vi "Initialize Hawkeye.vi"(0 "Repo / Workspace Folder Path":path, 1 "Generate Project for LVLib & Orphan Class":bool, 5 "LVLib / LVClass / Folder Path":path, 7 "Generate YAML Workflow from Template":bool, 9 "Generate Hawkeye Configuration from Template":bool, 12 "Generate .Hawkey File":bool) -> (4 "Status Indicator":string)   [LabVIEW 2019, in "HawkeyeToolsMenu.lvlib"]
doc: "GUI to compare LabVIEW code between currently checked out branch with any other branch or any of its commits.\n\n(c) 2024 Soliton Technologies. All rights reserved."
uses:
  HawkeyeToolsMenu.lvlib
  <vilib>/Hampel Software Engineering/Git API/Git API/GIT-api.lvclass
  <vilib>/Hampel Software Engineering/Git API/Git API/GIT-api.lvclass/GIT-api.ctl
  <vilib>/Hampel Software Engineering/Git API/Git API/Accessors/GIT-Set Working Dir.vi
  <userlib>/_OpenG.lib/file/file.llb/Valid Path - Traditional__ogtk.vi
  <userlib>/_OpenG.lib/file/file.llb/Compare Two Paths - Scalar__ogtk.vi
  <userlib>/_OpenG.lib/file/file.llb/File Exists - Scalar__ogtk.vi
  vi.lib/Hawkeye/Hawkeye.lvlib
panel:
  in  "Tab Control":enum32{"Main UI", "Help", "About"}(tab)
  in  "Generate HawkeyList":bool
  out "Current Status":string
  in  "Start Msg Indicator":string="Cofig Repo / Workspace Folder Path to Start"
  in  "Stop":bool
  in  "Start":bool
  # "1. Repository Path    -    Select the root folder where projects and configuration files will be created. Ensure the path is valid and accessible.\n\n2. Generation Options (Checkboxes) \n      Generate YAML Workflow from Template - Creates a YAML workflow file using a predefined template for automation or CI processes.\n      Generate Hawkeye Configuration from Template - Generates a Hawkeye configuration file based on a standard template for project setup.\n      Create Project for LVLib & Orphan Class - Creates LabVIEW project files (.lvproj) for each selected LVLib & Orphan LVClass.\n      Generate Hawkeye File - Creates a Hawkeye file specific to each project for build or analysis configuration.\n\n3. Start Button          -      Initiates the selected generation processes based on chosen options and updates status indicators.\n\n4. Status Indicators   -      Displays the progress of each selected operation, indicating whether it is pending, in progress, or completed."
  # "This tool automates the creation of LabVIEW project structures, including LVLibs, LVClasses, YAML workflows, and Hawkeye configuration files. It simplifies project setup by generating required files from predefined templates with minimal user input."
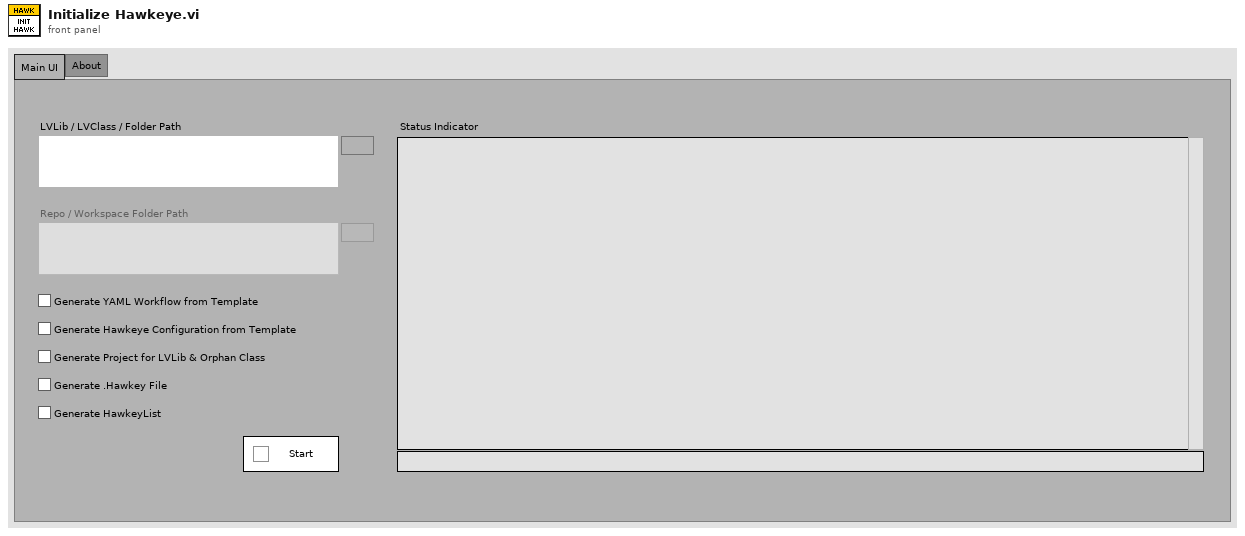
[diagram p1: front panel]
types:
  T1 = cluster{"Repository Path":path, "Git API Object":refnum<class "GIT-api.lvclass">, "Git API Initialized?":bool, "Generate YAML copy from template":bool, "Generate Cofig copy from template":bool, "Generate Project for LVLib":bool, "Generate Hawkey File":bool, "Generation Inprogress?":bool, "Status Indicator Ref":refnum<vi>, "BuildSpecsIncludePath":path, "LVLib / LVClass / Folder Path":path, "Current Status Ref":refnum<vi>, "Generate HawkeyList?":bool}
  T2 = enum8{"Enabled", "Disabled", "Disabled and Grayed Out"}
  T3 = typedef "Hawkeye.lvlib/HawkeyePathConfigs.ctl" = cluster{"GlobalIncludePaths":path[], "GlobalExcludePaths":path[], "BuildSpecsIncludePaths":path[], "ActualDepsIncludePaths":path[], "WorkspacePath":path, "SourceFolderPaths":path[], "ChangedFilesLogpaths":map{string, path}, "CacheRecreateDuration":dbl}
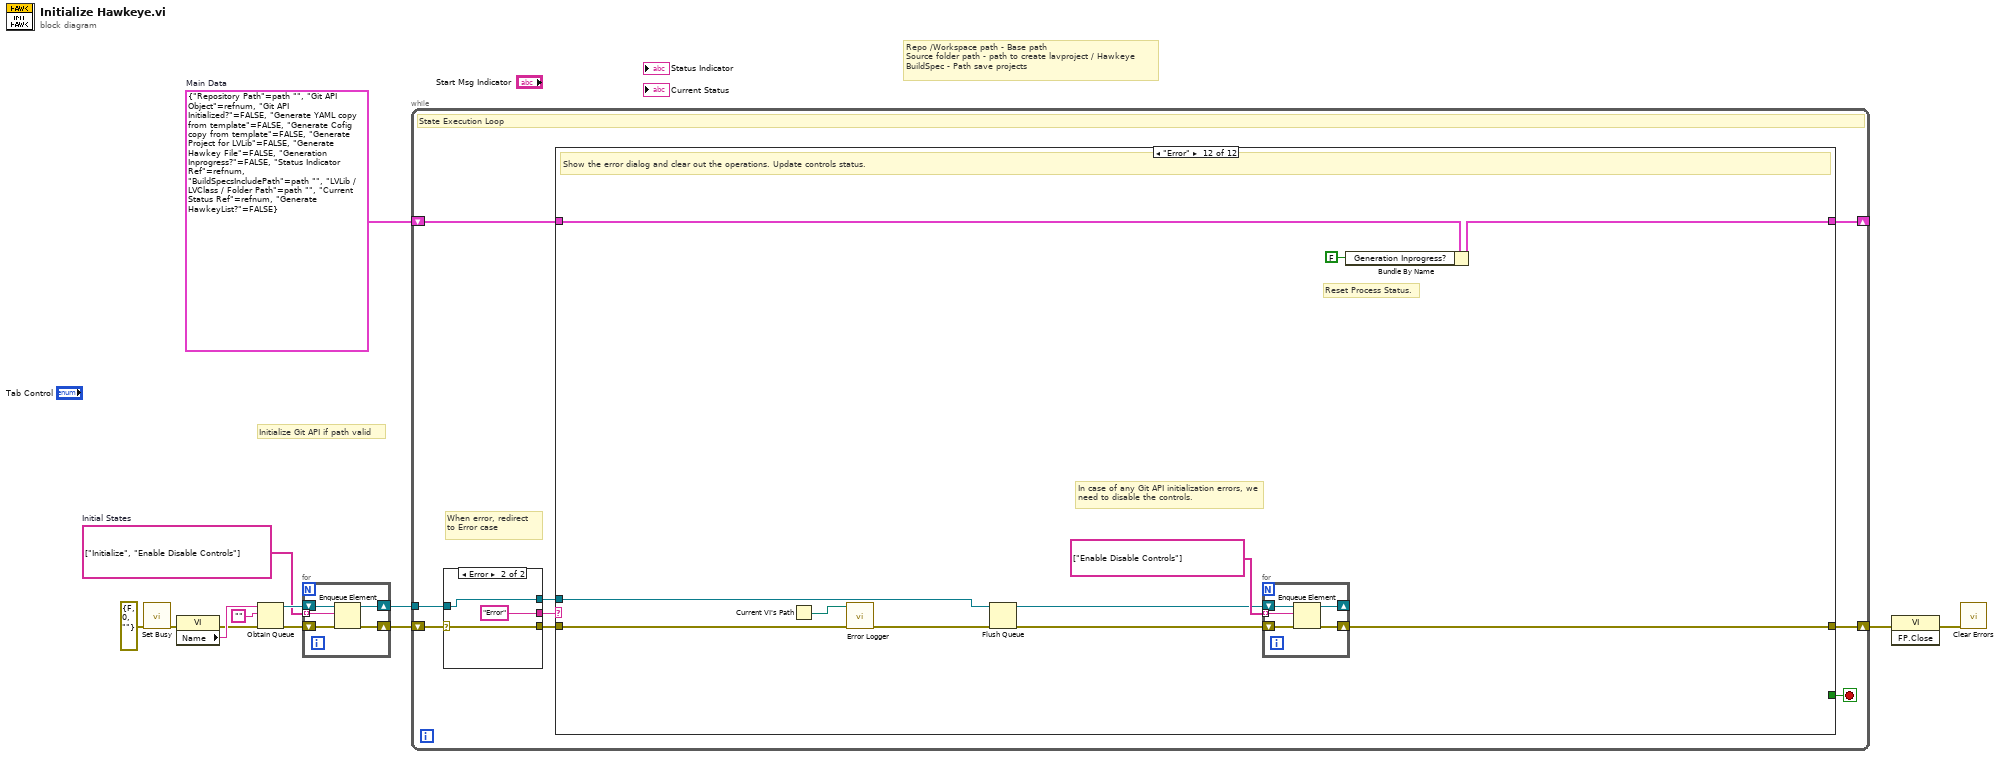
[diagram p0: block diagram]
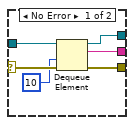
[diagram p2: hidden frame]
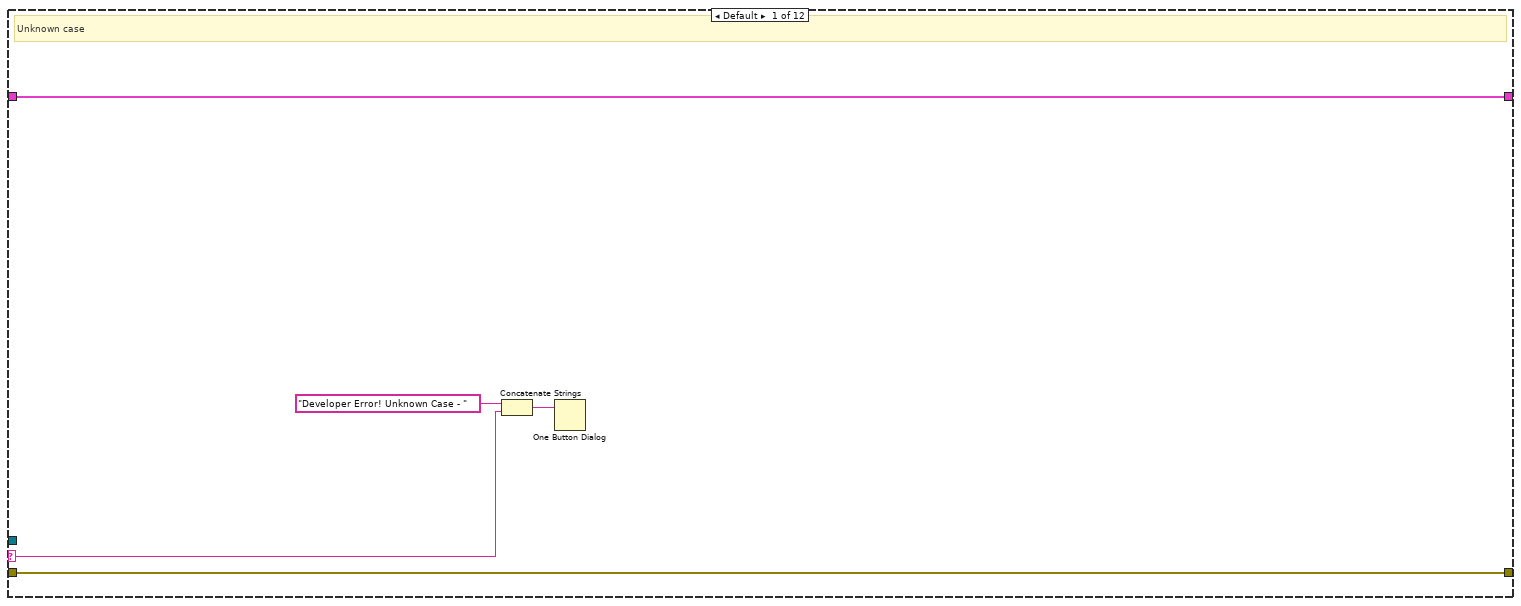
[diagram p3: hidden frame]
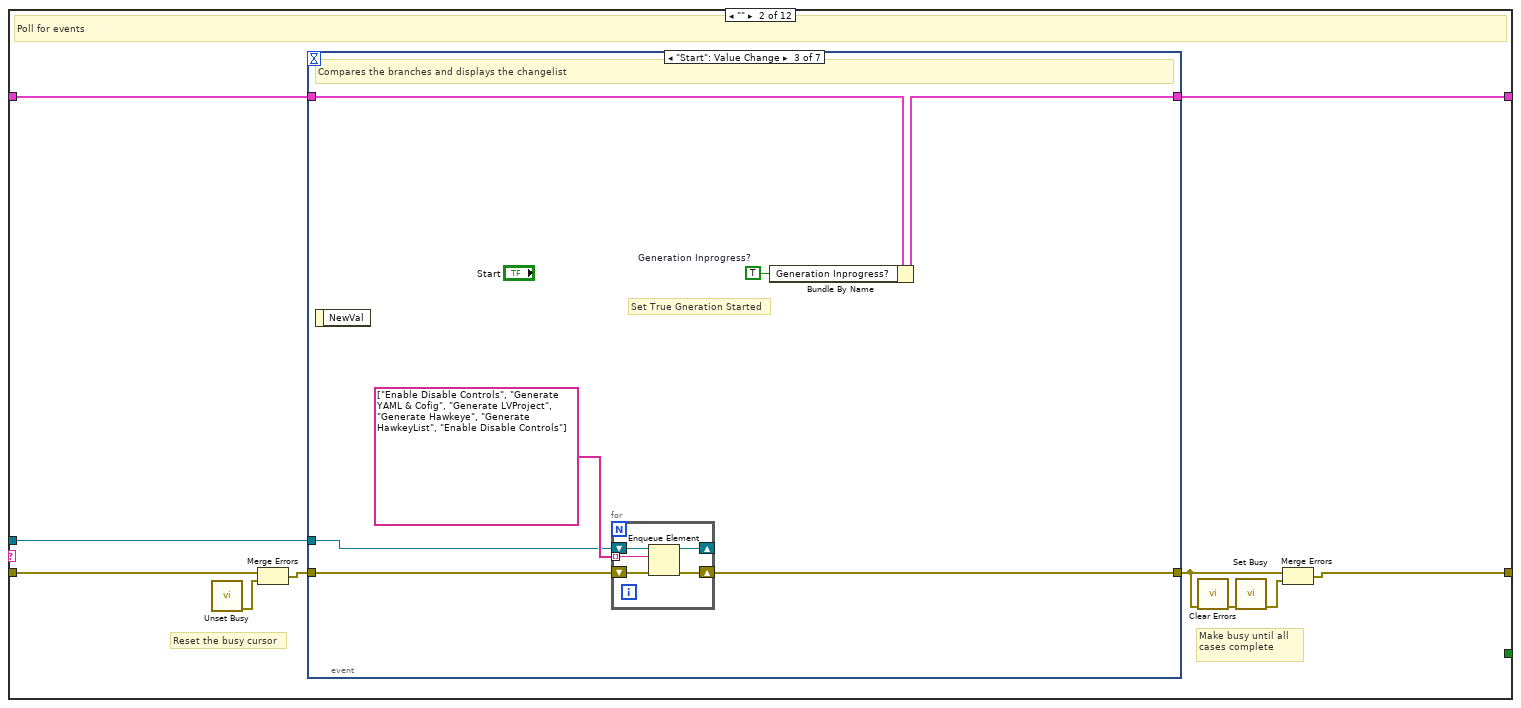
[diagram p4: hidden frame]
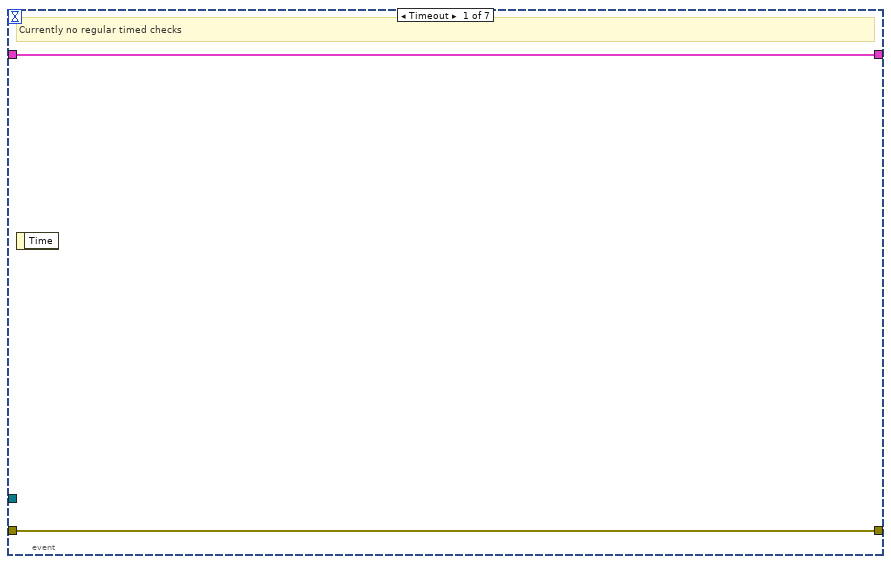
[diagram p5: hidden frame]
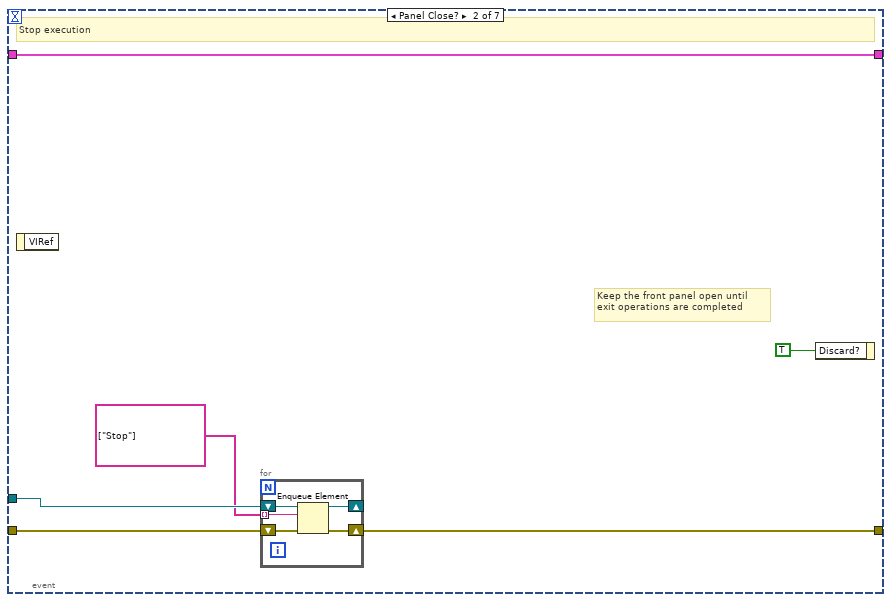
[diagram p6: hidden frame]
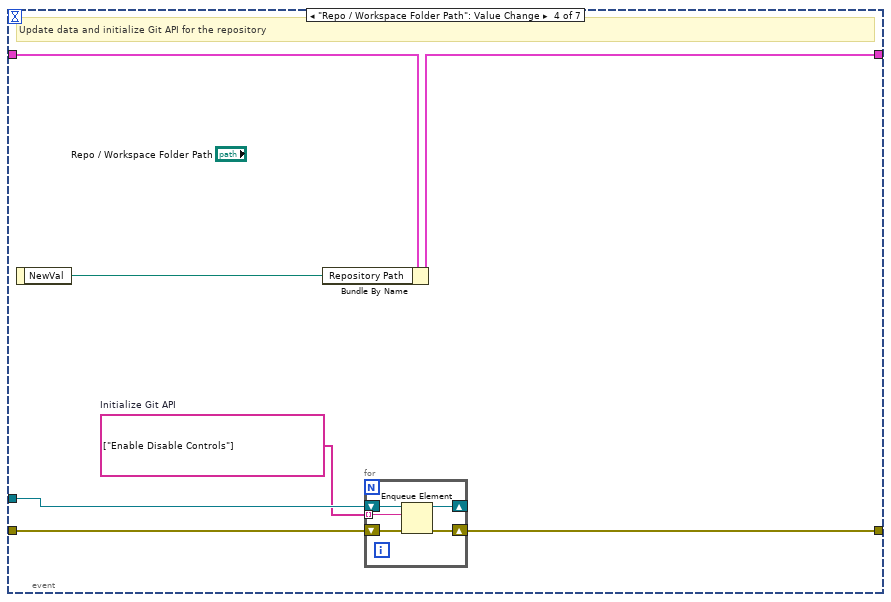
[diagram p7: hidden frame]
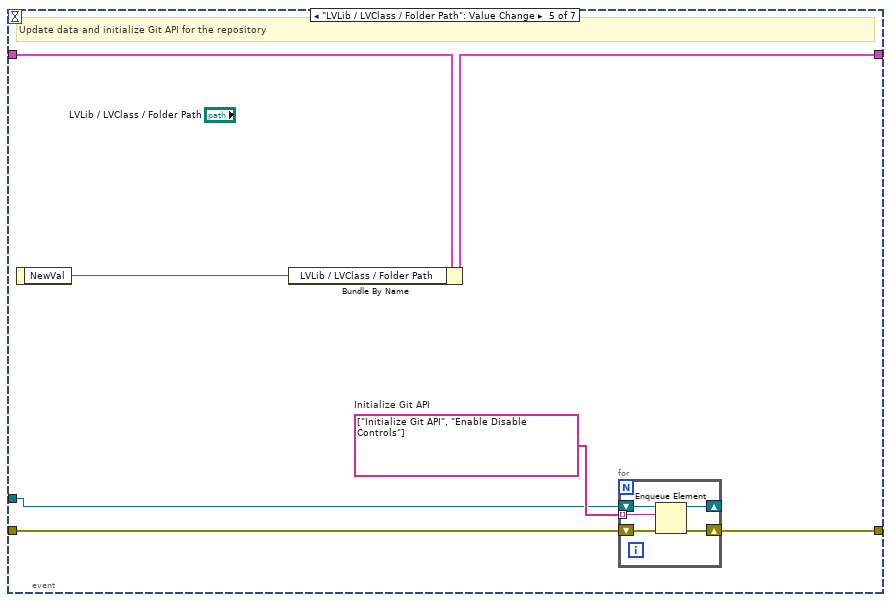
[diagram p8: hidden frame]
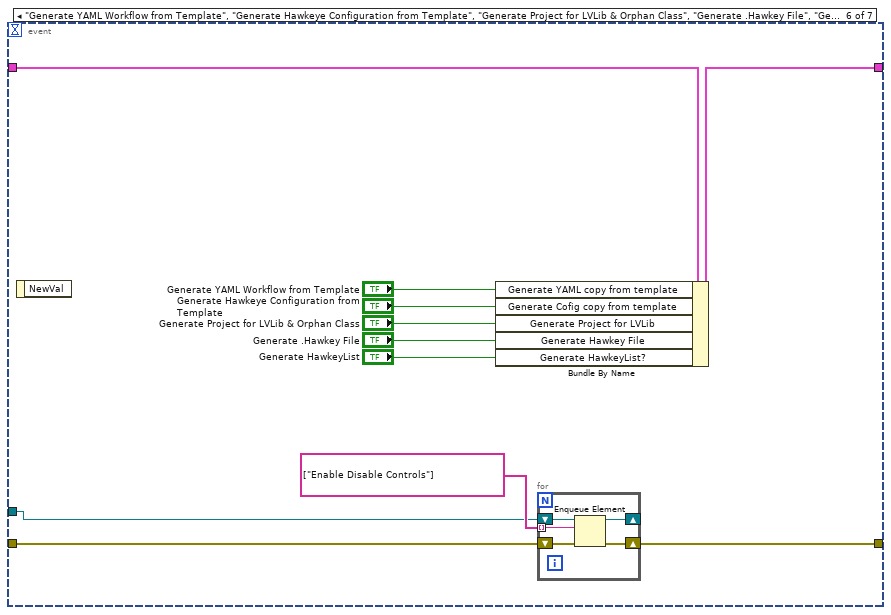
[diagram p9: hidden frame]
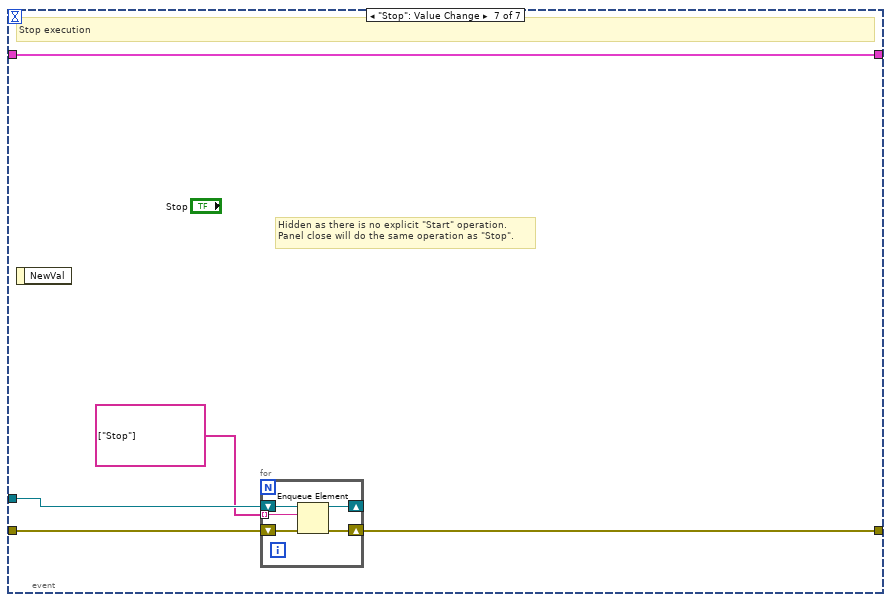
[diagram p10: hidden frame]
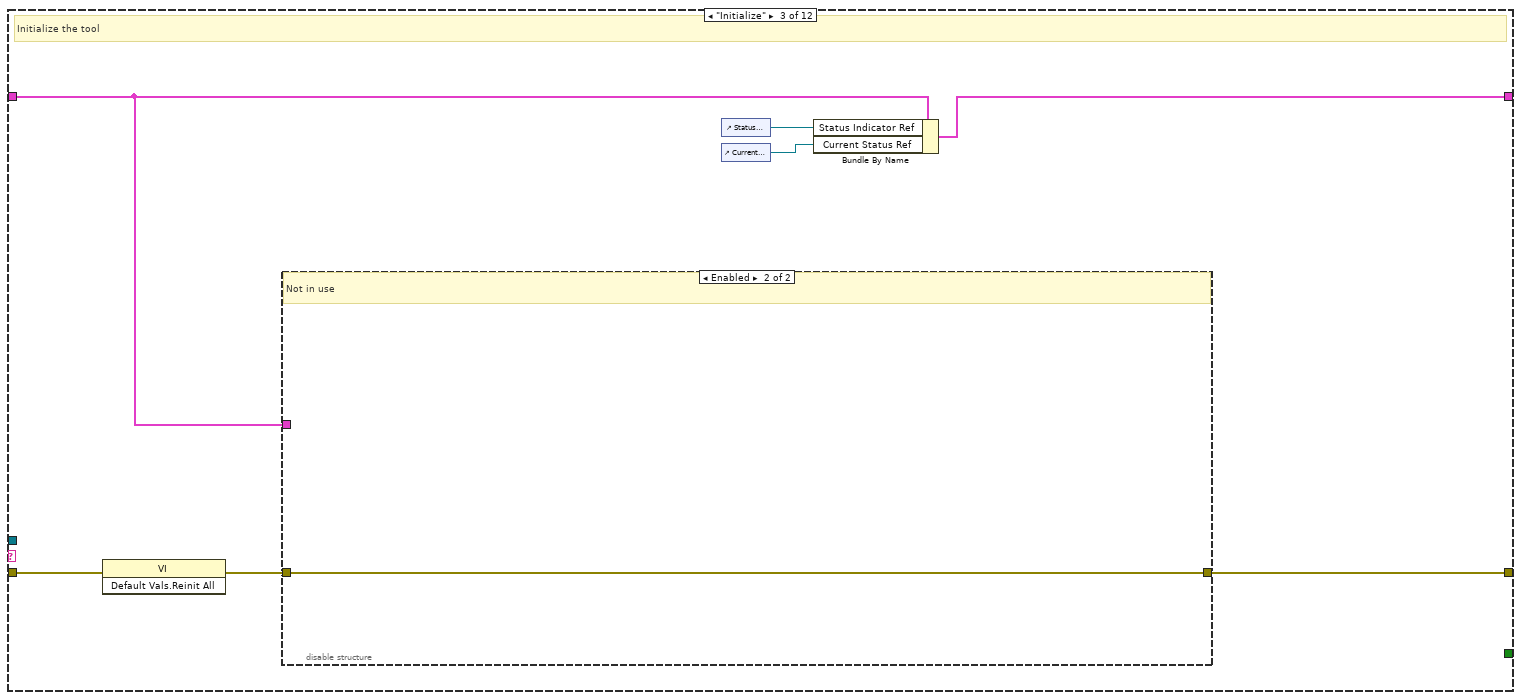
[diagram p11: hidden frame]
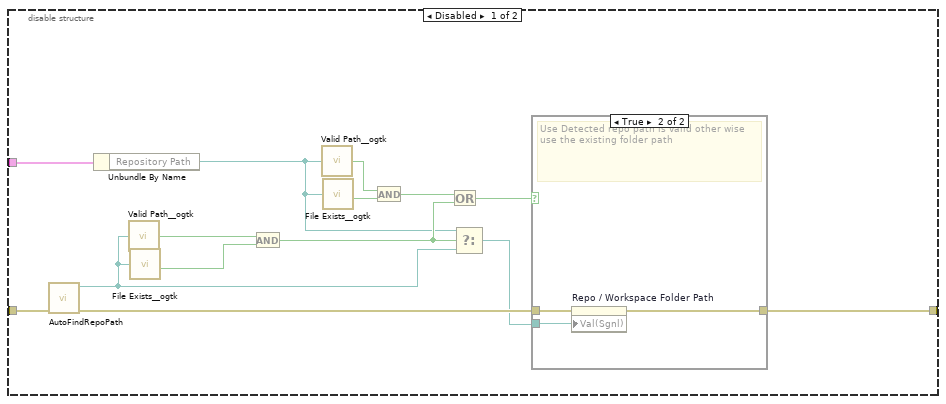
[diagram p12: hidden frame]
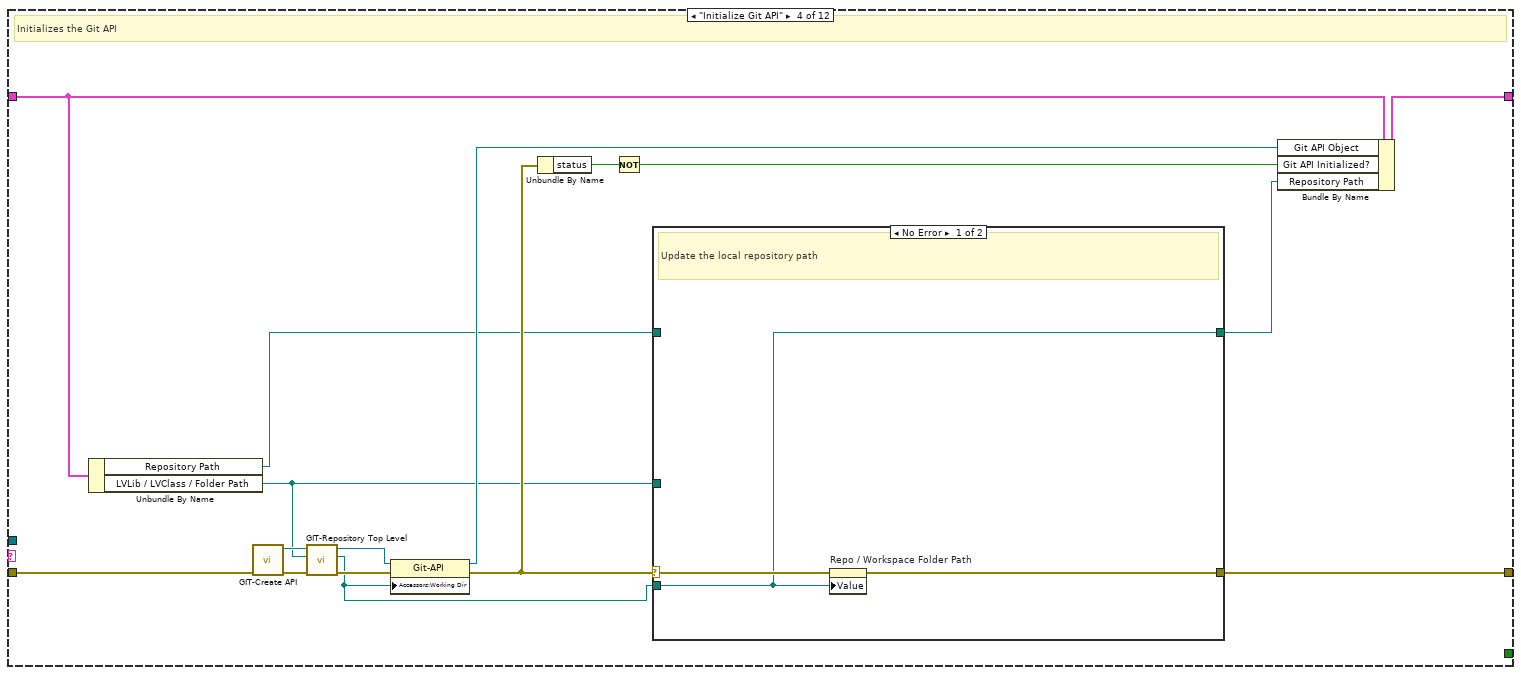
[diagram p14: hidden frame]
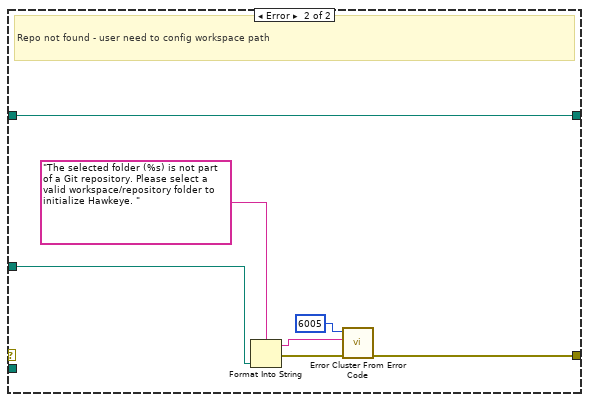
[diagram p15: hidden frame]
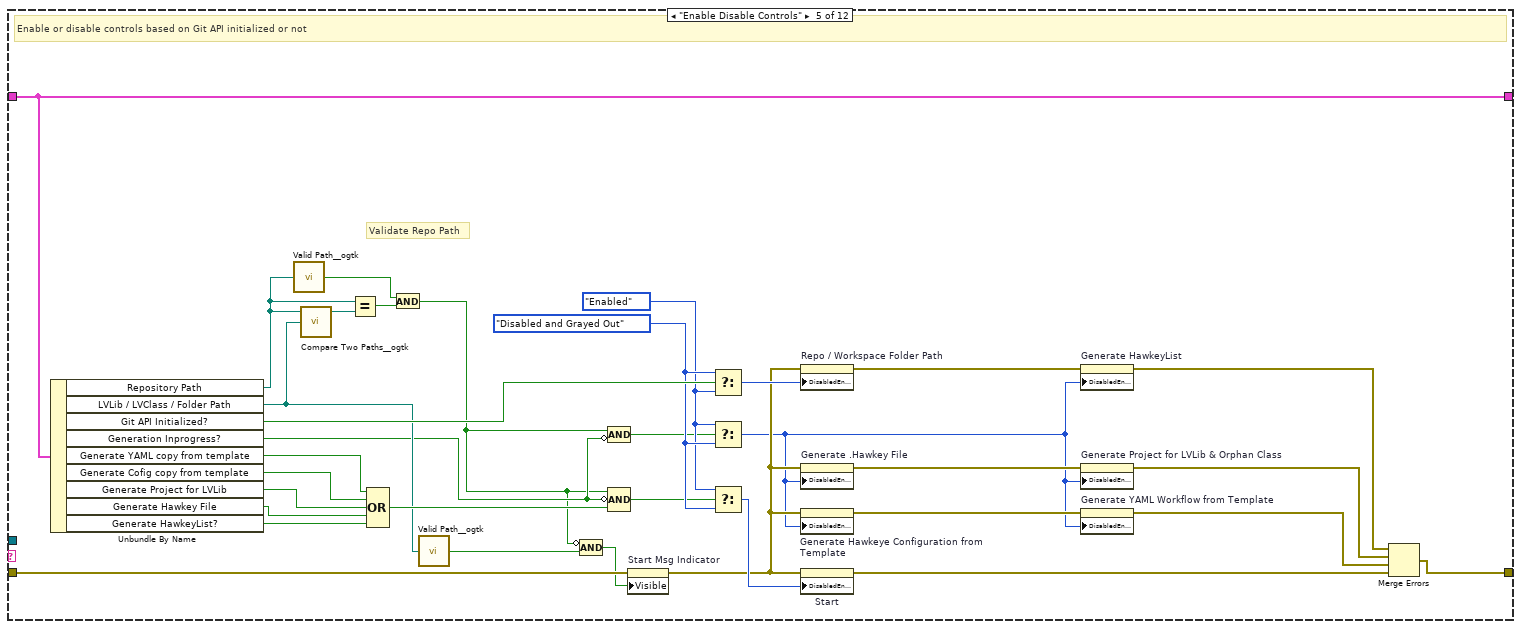
[diagram p16: hidden frame]
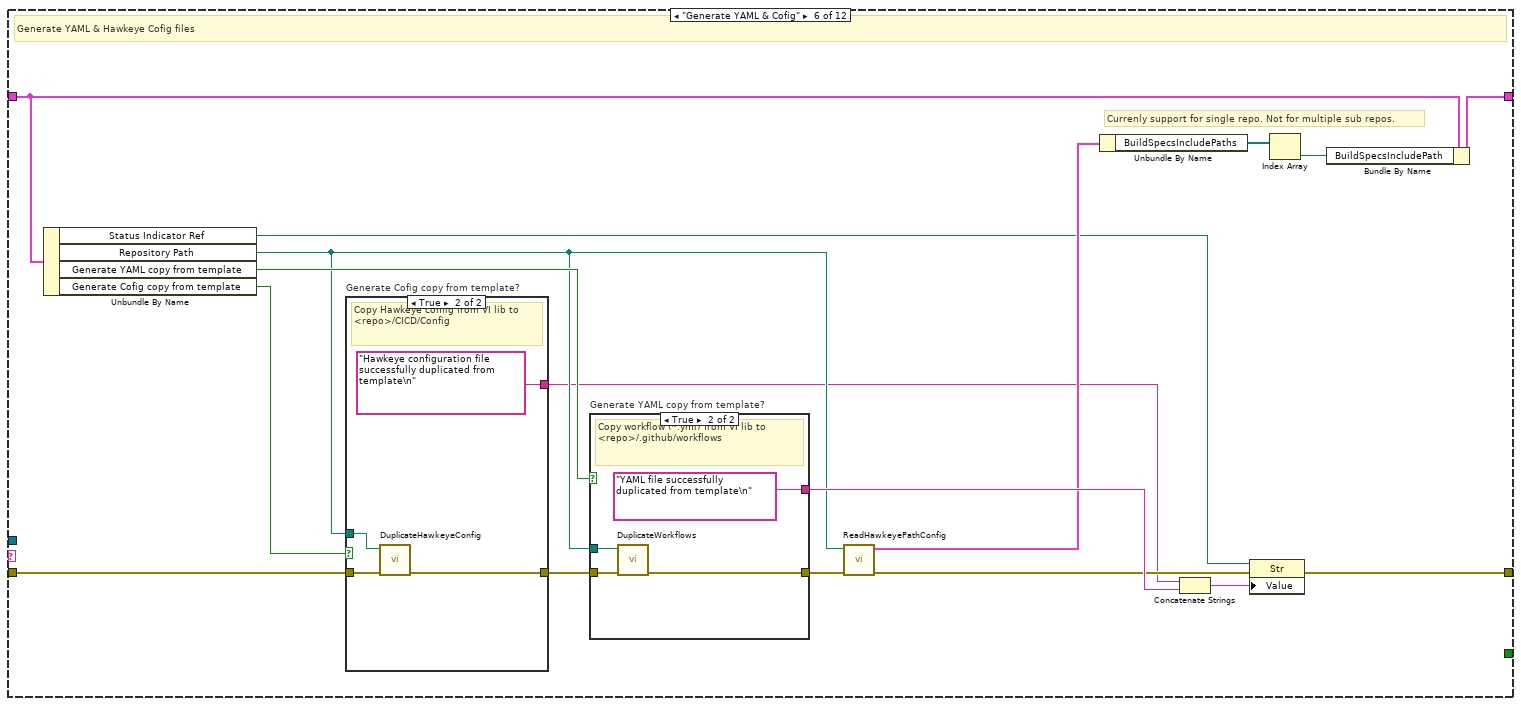
[diagram p17: hidden frame]
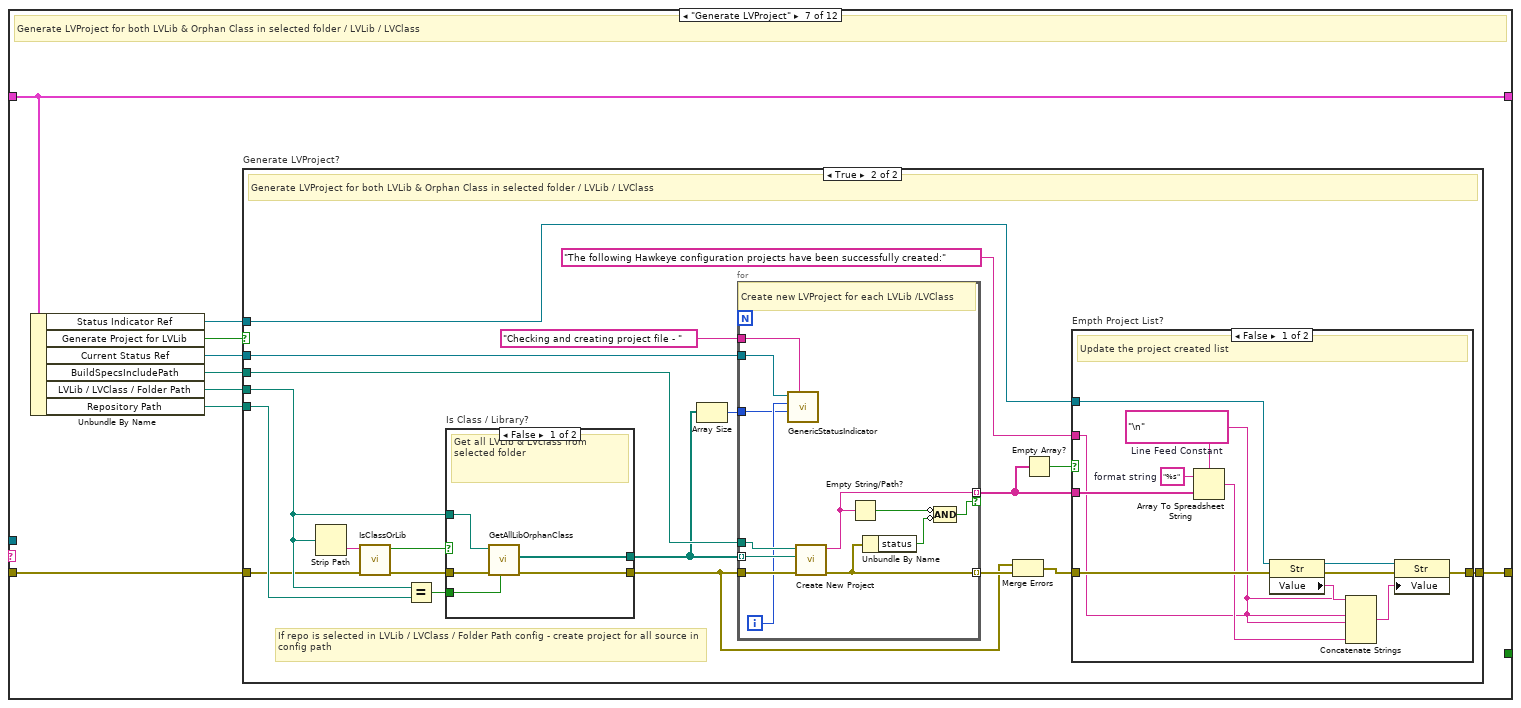
[diagram p20: hidden frame]
diagram:
  w1 = string[] ["Initialize", "Enable Disable Controls"]  # Initial States
  w10 = T1 {"Repository Path"=path "", "Git API Object"=refnum, "Git API Initialized?"=FALSE, "Generate YAML copy from template"=FALSE, "Generate Cofig copy from template"=FALSE, "Generate Project for LVLib"=FALSE, "Generate Hawkey File"=FALSE, "Generation Inprogress?"=FALSE, "Status Indicator Ref"=refnum, "BuildSpecsIncludePath"=path "", "LVLib / LVClass / Folder Path"=path "", "Current Status Ref"=refnum, "Generate HawkeyList?"=FALSE}  # Main Data
  # "Repo /Workspace path - Base path\nSource folder path - path to create lavproject / Hawkeye\nBuildSpec - Path save projects"
  # "Initialize Git API if path valid"
  n1 = call <vilib>:"Set Busy.vi"("error in (no error)"=errorcluster {"status"=FALSE, "code"=0, "source"=""}) -> ("error out"=w4:errorcluster)  [unwired: 9 in, 1 out]
  n2 = property class="VI"(error in=w4) -> (error out=w12:errorcluster, "Name"=w13:string)  [unwired: 1 in, 1 out]
  n3 = Obtain Queue(name (unnamed)=w13, element data type="", error in (no error)=w12) -> (queue out=w9:refnum<queue>, error out=w6:errorcluster)  [unwired: 2 in, 1 out]
  n4 = for {
    tunnel: w1 -> [w15] mode=indexing
    shift-right: [w17] -> w8
    shift-left: w6 -> [w18]
    shift-right: [w14] -> w7
    shift-left: w9 -> [w16]
    n5 = Enqueue Element(queue=w16, element=w15, error in (no error)=w18) -> (queue out=w14:refnum<queue>, error out=w17:errorcluster)  [unwired: 1 in, 1 out]
  }
  n6 = while {
    shift-right: [w19] -> w3
    shift-left: w8 -> [w21]
    tunnel: w7 -> [w22]
    shift-right: [w24] -> _
    shift-left: w10 -> [w23]
    stop <- w25 stop-if-true
    # "When error, redirect to Error case"
    # "State Execution Loop"
    n7 = case shown="Error" w21 {
      selector: w21 -> [w30 w34]
      tunnel: [w33 "Error" ("element")] -> w27
      tunnel: [w32 w36] -> w26
      tunnel: w22 -> [w31 w36]
      tunnel: [w28 w34] -> w20
      frame No Error {
        n8 = Dequeue Element(queue=w31, timeout in ms (-1)=10, error in (no error)=w30) -> (queue out=w32:refnum<queue>, element=w33:string, error out=w28:errorcluster)  [unwired: 1 out]
      }
      frame Error {
      }
    }
    n9 = case shown="\"Error\"" w27 {
      selector: w27 -> [w40 _ _ _ _ _ _ _ _ _ _ _]
      tunnel: w20 -> [w38 w45 w132 w168 w190 w228 w246 w308 w342 w357 w367 w370]
      tunnel: w26 -> [_ w51 _ _ _ _ _ _ _ w355 w364 w377]
      tunnel: [w38 w47 w131 w160 w195 w223 w247 w309 w343 w356 w363 w373] -> w19
      tunnel: [_ _ _ _ _ _ _ _ _ _ w365 _] -> w25
      tunnel: [w37 w49 w129 w166 w210 w220 w248 w310 w340 w354 w366 w372] -> w24
      tunnel: w23 -> [w37 w50 w128 w158 w210 w229 w248 w310 w344 w354 w366 w378]
      frame Default {
        # "Unknown case"
        n10 = Concatenate Strings("Developer Error! Unknown Case - " ("string"), w40) -> (w39:string)
        n11 = One Button Dialog(message=w39) -> ()  [unwired: 1 in, 1 out]
      }
      frame "" {
        # "Reset the busy cursor"
        # "Make busy until all cases complete"
        # "Poll for events"
        n12 = call <vilib>:"Unset Busy.vi"() -> ("error out"=w46:errorcluster)  [unwired: 11 in]
        n13 = Merge Errors(w45, w46) -> (w44:errorcluster)
        n14 = event shown="[2] \"Start\": Value Change" {
          selector: _ -> [_ _ _ _ _ _ _]
          dyn-events: _ -> [_ _ _ _ _ _ _]
          timeout: _ -> [_ _ _ _ _ _ _]
          tunnel: w44 -> [w52 w59 w70 w80 w89 w102 w121]
          tunnel: w51 -> [_ w58 w69 w79 w91 w104 w120]
          tunnel: [w52 w57 w68 w78 w90 w103 w119] -> w43
          tunnel: w50 -> [w53 w56 w67 w83 w95 w111 w118]
          tunnel: [w53 w56 w66 w82 w94 w110 w118] -> w49
          event Timeout {
            # "Currently no regular timed checks"
            n15 = event-data() -> ()  [unwired: 1 in, 1 out]
          }
          event Panel Close? {
            # "Keep the front panel open until exit operations are completed"
            # "Stop execution"
            n16 = event-data() -> ()  [unwired: 1 in, 1 out]
            n17 = for {
              tunnel: string[] ["Stop"] -> [w61] mode=indexing
              shift-right: [w63] -> w57
              shift-left: w59 -> [w64]
              shift-right: [w60] -> _
              shift-left: w58 -> [w62]
              n18 = Enqueue Element(queue=w62, element=w61, error in (no error)=w64) -> (queue out=w60:refnum<queue>, error out=w63:errorcluster)  [unwired: 1 in, 1 out]
            }
            n19 = event-data("Discard?"=TRUE) -> ()  [unwired: 1 in, 1 out]
          }
          event "Start": Value Change {
            w65 = TRUE  # Generation Inprogress?
            # "Set True Gneration Started"
            # "Compares the branches and displays the changelist"
            n20 = event-data() -> ()  [unwired: 1 in, 1 out]
            n21 = for {
              tunnel: string[] ["Enable Disable Controls", "Generate YAML & Cofig", "Generate LVProject", "Generate Hawkeye", "Generate HawkeyList", "Enable Disable Controls"] -> [w73] mode=indexing
              shift-right: [w75] -> w68
              shift-left: w70 -> [w76]
              shift-right: [w72] -> _
              shift-left: w69 -> [w74]
              n22 = Enqueue Element(queue=w74, element=w73, error in (no error)=w76) -> (queue out=w72:refnum<queue>, error out=w75:errorcluster)  [unwired: 1 in, 1 out]
            }
            n23 = Bundle By Name(cluster=w67, "Generation Inprogress?"=w65) -> (w66:T1)
          }
          event "Repo / Workspace Folder Path": Value Change {
            w77 = string[] ["Enable Disable Controls"]  # Initialize Git API
            # "Update data and initialize Git API for the repository"
            n24 = event-data() -> ("NewVal"=w81:path)  [unwired: 1 in]
            n25 = Bundle By Name(cluster=w83, "Repository Path"=w81) -> (w82:T1)
            n26 = for {
              tunnel: w77 -> [w85] mode=indexing
              shift-right: [w87] -> w78
              shift-left: w80 -> [w88]
              shift-right: [w84] -> _
              shift-left: w79 -> [w86]
              n27 = Enqueue Element(queue=w86, element=w85, error in (no error)=w88) -> (queue out=w84:refnum<queue>, error out=w87:errorcluster)  [unwired: 1 in, 1 out]
            }
          }
          event "LVLib / LVClass / Folder Path": Value Change {
            w92 = string[] ["Initialize Git API", "Enable Disable Controls"]  # Initialize Git API
            # "Update data and initialize Git API for the repository"
            n28 = event-data() -> ("NewVal"=w93:path)  [unwired: 1 in]
            n29 = Bundle By Name(cluster=w95, "LVLib / LVClass / Folder Path"=w93) -> (w94:T1)
            n30 = for {
              tunnel: w92 -> [w97] mode=indexing
              shift-right: [w99] -> w90
              shift-left: w89 -> [w100]
              shift-right: [w96] -> _
              shift-left: w91 -> [w98]
              n31 = Enqueue Element(queue=w98, element=w97, error in (no error)=w100) -> (queue out=w96:refnum<queue>, error out=w99:errorcluster)  [unwired: 1 in, 1 out]
            }
          }
          event "Generate YAML Workflow from Template", "Generate Hawkeye Configuration from Template", "Generate Project for LVLib & Orphan Class", "Generate .Hawkey File", "Generate HawkeyList": Value Change {
            n32 = event-data() -> ()  [unwired: 1 in, 1 out]
            n33 = Bundle By Name(cluster=w111, "Generate YAML copy from template"="Generate YAML Workflow from Template", "Generate Cofig copy from template"="Generate Hawkeye Configuration from Template", "Generate Project for LVLib"="Generate Project for LVLib & Orphan Class", "Generate Hawkey File"="Generate .Hawkey File", "Generate HawkeyList?"="Generate HawkeyList") -> (w110:T1)
            n34 = for {
              tunnel: string[] ["Enable Disable Controls"] -> [w113] mode=indexing
              shift-right: [w115] -> w103
              shift-left: w102 -> [w116]
              shift-right: [w112] -> _
              shift-left: w104 -> [w114]
              n35 = Enqueue Element(queue=w114, element=w113, error in (no error)=w116) -> (queue out=w112:refnum<queue>, error out=w115:errorcluster)  [unwired: 1 in, 1 out]
            }
          }
          event "Stop": Value Change {
            # "Hidden as there is no explicit \"Start\" operation.\nPanel close will do the same operation as \"Stop\"."
            # "Stop execution"
            n36 = event-data() -> ()  [unwired: 1 in, 1 out]
            n37 = for {
              tunnel: string[] ["Stop"] -> [w123] mode=indexing
              shift-right: [w125] -> w119
              shift-left: w121 -> [w126]
              shift-right: [w122] -> _
              shift-left: w120 -> [w124]
              n38 = Enqueue Element(queue=w124, element=w123, error in (no error)=w126) -> (queue out=w122:refnum<queue>, error out=w125:errorcluster)  [unwired: 1 in, 1 out]
            }
          }
        }
        n39 = call <vilib>:"Clear Errors.vi"("error in (no error)"=w43) -> ("error out"=w42:errorcluster)  [unwired: 5 in, 1 out]
        n40 = call <vilib>:"Set Busy.vi"("error in (no error)"=w42) -> ("error out"=w48:errorcluster)  [unwired: 9 in, 1 out]
        n41 = Merge Errors(w43, w48) -> (w47:errorcluster)
      }
      frame "Initialize" {
        # "Initialize the tool"
        n42 = invoke class="VI" method="Default Vals.Reinit All"(error in=w132) -> (error out=w133:errorcluster)  [unwired: 2 in, 2 out]
        n43 = disable-structure shown="Enabled" {
          disable-tunnel: w128 -> [w144 _]
          disable-tunnel: w133 -> [w137 w152]
          disable-tunnel: [w136 w152] -> w131
          frame Disabled {
            n44 = call "AutoFindRepoPath.vi"("error in (no error)"=w137) -> ("error out"=w147:errorcluster, "Repo Path"=w135:path)  [unwired: 9 in]
            n45 = Unbundle By Name(w144) -> ("Repository Path"=w134:path)
            n46 = call-poly <userlib>:"Valid Path__ogtk.vi"("path"=w135) -> ("valid"=w145:bool)
            n47 = call-poly <userlib>:"File Exists__ogtk.vi"("file path"=w135) -> ("exists"=w146:bool)  [unwired: 6 in, 1 out]
            n48 = And(x=w145, y=w146) -> (x .and. y?=w138:bool)
            n49 = call-poly <userlib>:"Valid Path__ogtk.vi"("path"=w134) -> ("valid"=w140:bool)
            n50 = call-poly <userlib>:"File Exists__ogtk.vi"("file path"=w134) -> ("exists"=w143:bool)  [unwired: 6 in, 1 out]
            n51 = And(x=w140, y=w143) -> (x .and. y?=w142:bool)
            n52 = Or(x=w142, y=w138) -> (x .or. y?=w141:bool)
            n53 = Select(t=w134, s=w138, f=w135) -> (s? t:f=w139:path)
            n54 = case shown="True" w141 {
              tunnel: w147 -> [w148 w151]
              tunnel: [w148 w149] -> w136
              tunnel: w139 -> [_ w150]
              frame False {
              }
              frame True {
                # "Use Detected repo path is valid other wise use the existing folder path"
                n55 = property on="Repo / Workspace Folder Path" class="Path"(error in=w151, "Val(Sgnl)"=w150) -> (error out=w149:errorcluster)  [unwired: 1 in, 1 out]
              }
            }
          }
          frame Enabled {
            # "Not in use"
          }
        }
        n56 = control-ref of="Status Indicator Ref"() -> (w130:refnum<vi>)
        n57 = control-ref of="Current Status"() -> (w127:refnum<vi>)
        n58 = Bundle By Name(cluster=w128, "Status Indicator Ref"=w130, "Current Status Ref"=w127) -> (w129:T1)
      }
      frame "Initialize Git API" {
        # "Initializes the Git API"
        n59 = Unbundle By Name(w158) -> ("Repository Path"=w153:path, "LVLib / LVClass / Folder Path"=w155:path)
        n60 = call <vilib>:"GIT-Create API.vi"("error in"=w168) -> ("error out"=w165:errorcluster, "git-api out"=w163:refnum<class "GIT-api.lvclass">)  [unwired: 9 in]
        n61 = call <vilib>:"GIT-Repository Top Level.vi"("error in"=w165, "Current Path"=w155, "git-api in"=w163) -> ("error out"=w162:errorcluster, "Repo Top Level Path"=w156:path, "git-api out"=w164:refnum<class "GIT-api.lvclass">)  [unwired: 6 in]
        n62 = property class="Git-API"(reference=w164, error in=w162, "Accessors:Working Dir"=w156) -> (reference out=w167:refnum<class "GIT-api.lvclass">, error out=w157:errorcluster)
        n63 = Unbundle By Name(w157) -> ("status"=w161:bool)
        n64 = Not(x=w161) -> (.not. x?=w159:bool)
        n65 = case shown="No Error" w157 {
          selector: w157 -> [w170 _]
          tunnel: [w171 w174] -> w160
          tunnel: w156 -> [w169 _]
          tunnel: w155 -> [_ w173]
          tunnel: [w169 w172] -> w154
          tunnel: w153 -> [_ w172]
          frame No Error {
            # "Update the local repository path"
            n66 = property on="Repo / Workspace Folder Path" class="Path"(error in=w170, "Value"=w169) -> (error out=w171:errorcluster)  [unwired: 1 in, 1 out]
          }
          frame Error {
            # "Repo not found - user need to config workspace path"
            n67 = Format Into String(format string="The selected folder (%s) is not part of a Git repository. Please select a valid workspace/repository folder to initialize Hawkeye. ", w173) -> (resulting string=w175:string, error out=w178:errorcluster)  [unwired: 2 in]
            n68 = call <vilib>:"Error Cluster From Error Code.vi"("error in (no error)"=w178, "error message (\"\")"=w175, "error code (0)"=6005) -> ("error out"=w174:errorcluster)  [unwired: 6 in]
          }
        }
        n69 = Bundle By Name(cluster=w158, "Git API Object"=w167, "Git API Initialized?"=w159, "Repository Path"=w154) -> (w166:T1)
      }
      frame "Enable Disable Controls" {
        w200 = T2."Disabled and Grayed Out" ("Disabled")
        w199 = T2."Enabled" ("Disabled")
        # "Validate Repo Path"
        # "Enable or disable controls based on Git API initialized or not"
        n70 = Unbundle By Name(w210) -> ("Repository Path"=w205:path, "LVLib / LVClass / Folder Path"=w189:path, "Git API Initialized?"=w201:bool, "Generation Inprogress?"=w184:bool, "Generate YAML copy from template"=w212:bool, "Generate Cofig copy from template"=w211:bool, "Generate Project for LVLib"=w209:bool, "Generate Hawkey File"=w208:bool, "Generate HawkeyList?"=w179:bool)
        n71 = call-poly <userlib>:"Valid Path__ogtk.vi"("path"=w205) -> ("valid"=w204:bool)
        n72 = call-poly <userlib>:"Compare Two Paths__ogtk.vi"("path2"=w189, "path1"=w205) -> ("common path"=w207:path)  [unwired: 1 in, 2 out]
        n73 = Equal?(x=w205, y=w207) -> (x = y?=w206:bool)
        n74 = Compound Arithmetic op=OR(w212, w211, w209, w208, w179) -> (w203:bool)
        n75 = And(x=w204, y=w206) -> (x .and. y?=w183:bool)
        n76 = call-poly <userlib>:"Valid Path__ogtk.vi"("path"=w189) -> ("valid"=w188:bool)
        n77 = Compound Arithmetic op=AND(invert w183, w188) -> (w186:bool)
        n78 = Compound Arithmetic op=AND(w183, invert w184) -> (w185:bool)
        n79 = Compound Arithmetic op=AND(w183, invert w184, w203) -> (w187:bool)
        n80 = property on="Start Msg Indicator" class="Str"(error in=w190, "Visible"=w186) -> (error out=w191:errorcluster)  [unwired: 1 in, 1 out]
        n81 = Select(t=w200, s=w201, f=w199) -> (s? t:f=w198:T2)
        n82 = Select(t=w199, s=w185, f=w200) -> (s? t:f=w180:T2)
        n83 = Select(t=w199, s=w187, f=w200) -> (s? t:f=w202:T2)
        n84 = property on="Repo / Workspace Folder Path" class="Path"(error in=w191, "DisabledEnum"=w198) -> (error out=w182:errorcluster)  [unwired: 1 in, 1 out]
        n85 = property on="Generate .Hawkey File" class="Bool (strict)"(error in=w191, "DisabledEnum"=w180) -> (error out=w197:errorcluster)  [unwired: 1 in, 1 out]
        n86 = property on="Generate Hawkeye Configuration from Template" class="Bool (strict)"(error in=w191, "DisabledEnum"=w180) -> (error out=w196:errorcluster)  [unwired: 1 in, 1 out]
        n87 = property on="Start" class="Bool"(error in=w191, "DisabledEnum"=w202) -> (error out=w194:errorcluster)  [unwired: 1 in, 1 out]
        n88 = property on="Generate HawkeyList" class="Bool (strict)"(error in=w182, "DisabledEnum"=w180) -> (error out=w181:errorcluster)  [unwired: 1 in, 1 out]
        n89 = property on="Generate Project for LVLib & Orphan Class" class="Bool (strict)"(error in=w197, "DisabledEnum"=w180) -> (error out=w192:errorcluster)  [unwired: 1 in, 1 out]
        n90 = property on="Generate YAML Workflow from Template" class="Bool (strict)"(error in=w196, "DisabledEnum"=w180) -> (error out=w193:errorcluster)  [unwired: 1 in, 1 out]
        n91 = Merge Errors(w181, w192, w193, w194) -> (w195:errorcluster)
      }
      frame "Generate YAML & Cofig" {
        # "Currenly support for single repo. Not for multiple sub repos."
        # "Generate YAML & Hawkeye Cofig files"
        n92 = Unbundle By Name(w229) -> ("Status Indicator Ref"=w218:refnum<vi>, "Repository Path"=w219:path, "Generate YAML copy from template"=w226:bool, "Generate Cofig copy from template"=w227:bool)
        n93 = case "Generate Cofig copy from template?" shown="True" w227 {
          tunnel: [w235 w236] -> w216
          tunnel: w219 -> [_ w238]
          tunnel: w228 -> [w235 w237]
          tunnel: [_ "Hawkeye configuration file successfully duplicated from template\n"] -> w217
          frame False {
            # "Skip Generate Cofig copy from template"
          }
          frame True {
            # "Copy Hawkeye config from VI lib to <repo>/CICD/Config"
            n94 = call "DuplicateHawkeyeConfig.vi"("error in (no error)"=w237, "Repo / Workspace Folder Path"=w238) -> ("error out"=w236:errorcluster)  [unwired: 9 in]
          }
        }
        n95 = case "Generate YAML copy from template?" shown="True" w226 {
          tunnel: w219 -> [_ w233]
          tunnel: [w230 w231] -> w215
          tunnel: w216 -> [w230 w232]
          tunnel: [_ "YAML file successfully duplicated from template\n"] -> w225
          frame False {
            # "Skip Generate YAML copy from template"
          }
          frame True {
            # "Copy workflow (*.yml) from VI lib to <repo>/.github/workflows"
            n96 = call "DuplicateWorkflows.vi"("error in (no error)"=w232, "Repo / Workspace Folder Path"=w233) -> ("error out"=w231:errorcluster)  [unwired: 9 in]
          }
        }
        n97 = call "ReadHawkeyePathConfig.vi"("error in (no error)"=w215, "Workspace Path"=w219) -> ("error out"=w221:errorcluster, "Hawkeye Path Config Out"=w222:T3)  [unwired: 8 in]
        n98 = Unbundle By Name(w222) -> ("BuildSpecsIncludePaths"=w214:path[])
        n99 = Concatenate Strings(w217, w225) -> (w224:string)
        n100 = property class="Str"(reference=w218, error in=w221, "Value"=w224) -> (error out=w223:errorcluster)  [unwired: 1 out]
        n101 = Index Array(array=w214) -> (element=w213:path)  [unwired: 1 in]
        n102 = Bundle By Name(cluster=w229, "BuildSpecsIncludePath"=w213) -> (w220:T1)
      }
      frame "Generate LVProject" {
        # "Generate LVProject for both LVLib & Orphan Class in selected folder / LVLib / LVClass"
        n103 = Unbundle By Name(w248) -> ("Status Indicator Ref"=w241:refnum<vi>, "Generate Project for LVLib"=w240:bool, "Current Status Ref"=w244:refnum<vi>, "BuildSpecsIncludePath"=w245:path, "LVLib / LVClass / Folder Path"=w243:path, "Repository Path"=w242:path)
        n104 = case "Generate LVProject?" shown="True" w240 {
          tunnel: [w249 w253] -> w247
          tunnel: w246 -> [w249 w258]
          tunnel: w245 -> [_ w263]
          tunnel: w244 -> [_ w268]
          tunnel: w243 -> [_ w261]
          tunnel: w242 -> [_ w262]
          tunnel: w241 -> [_ w254]
          frame False {
            # "Skipped LVProject reaction"
          }
          frame True {
            # "If repo is selected in LVLib / LVClass / Folder Path config - create project for all source in config path"
            # "Generate LVProject for both LVLib & Orphan Class in selected folder / LVLib / LVClass"
            n105 = Strip Path(path=w261) -> (name=w267:string)  [unwired: 1 out]
            n106 = call "IsClassOrLib.vi"("error in (no error)"=w258, "LVFile Name"=w267) -> ("error out"=w259:errorcluster, "Is LVClass or Library?"=w265:bool)  [unwired: 8 in]
            n107 = Equal?(x=w261, y=w262) -> (x = y?=w260:bool)
            n108 = case "Is Class / Library?" shown="False" w265 {
              tunnel: w259 -> [w287 w290]
              tunnel: w261 -> [w286 w289]
              tunnel: [w285 w290] -> w264
              tunnel: [w284 w288] -> w257
              tunnel: w260 -> [w283 _]
              frame False {
                # "Get all LVLib & LVclass from selected folder"
                n109 = call "GetAllLibOrphanClass.vi"("Get From All Src Folder?"=w283, "error in (no error)"=w287, "Workspace Path"=w286) -> ("error out"=w285:errorcluster, "Lib / Class Path []"=w284:path[])  [unwired: 6 in, 1 out]
              }
              frame True {
                # "Create project for selected Class / Lib"
                n110 = Build Array(w289) -> (w288:path[])
              }
            }
            n111 = Array Size(array=w257) -> (size(s)=w256:i32)
            n112 = for {
              tunnel: w263 -> [w301]
              tunnel: w257 -> [w300] mode=indexing
              tunnel: w264 -> [w302]
              tunnel: [w294] -> w266 mode=indexing
              tunnel: w268 -> [w299]
              tunnel: w256 -> [w297]
              tunnel: "Checking and creating project file - " ("Prefix to append") -> [w296]
              tunnel: [w295] -> w252 mode=indexing if=w291
              i -> [w298]
              # "Create new LVProject for each LVLib /LVClass"
              n113 = call "GenericStatusIndicator.vi"("Prefix to append"=w296, "Total"=w297, "Current Iteration"=w298, "Status Indicator Ref In"=w299) -> ()  [unwired: 7 in, 1 out]
              n114 = call "Create New Project.vi"("error in (no error)"=w302, "File Path to Append"=w300, "Build Specs Folder Path"=w301) -> ("error out"=w294:errorcluster, "Project Created"=w295:string)  [unwired: 7 in]
              n115 = Empty String/Path?(string/path=w295) -> (empty?=w293:bool)
              n116 = Unbundle By Name(w294) -> ("status"=w292:bool)
              n117 = Compound Arithmetic op=AND(invert w293, invert w292) -> (w291:bool)
            }
            n118 = Merge Errors(w264, w266) -> (w269:errorcluster)
            n119 = Empty Array?(array=w252) -> (empty?=w251:bool)
            n120 = case "Empth Project List?" shown="False" w251 {
              tunnel: w269 -> [w281 w282]
              tunnel: w254 -> [w279 _]
              tunnel: [w278 w282] -> w253
              tunnel: w252 -> [w274 _]
              tunnel: "The following Hawkeye configuration projects have been successfully created:" ("string") -> [w271 _]
              frame False {
                w270 = "\n"  # Line Feed Constant
                w273 = "%s"  # format string
                # "Update the project created list"
                n121 = Array To Spreadsheet String(delimiter (Tab)=w270, array=w274, 3:w273) -> (spreadsheet string=w272:string)
                n122 = property class="Str"(reference=w279, error in=w281) -> (reference out=w276:refnum<vi>, error out=w280:errorcluster, "Value"=w277:string)
                n123 = Concatenate Strings(w277, w270, w271, w270, w270, w272) -> (w275:string)
                n124 = property class="Str"(reference=w276, error in=w280, "Value"=w275) -> (error out=w278:errorcluster)  [unwired: 1 out]
              }
              frame True {
                # "No need to update any status"
              }
            }
          }
        }
      }
      frame "Generate Hawkeye" {
        # "Create new .Hawkeye files"
        n125 = Unbundle By Name(w310) -> ("Status Indicator Ref"=w303:refnum<vi>, "Current Status Ref"=w305:refnum<vi>, "Generate Hawkey File"=w307:bool, "Repository Path"=w304:path, "LVLib / LVClass / Folder Path"=w306:path)
        n126 = case "Generate Hawkey File ?" shown="True" w307 {
          tunnel: [w311 w317] -> w309
          tunnel: w308 -> [w311 w322]
          tunnel: w306 -> [_ w321]
          tunnel: w305 -> [_ w314]
          tunnel: w304 -> [_ w320]
          tunnel: w303 -> [_ w315]
          frame False {
            # "Skipped Generate .Hawkey"
          }
          frame True {
            w319 = FALSE  # Check Changed Libraries Only?
            # "During Initial creation check all items in selected folder/path"
            # "Generate Hawkey File for selected LVLib / LVClass / Folder"
            n127 = call "Generate Hawkeye File.vi"("Status Indicator Ref"=w314, "error in (no error)"=w322, "Check Changed Libraries Only?"=w319, "LVLib / LVClass / Folder Path"=w321, "Repo Folder Path"=w320) -> ("error out"=w318:errorcluster, ".hawkeye created"=w313:string[])  [unwired: 5 in]
            n128 = Empty Array?(array=w313) -> (empty?=w312:bool)
            n129 = case "Empth hawkeye List?" shown="False" w312 {
              tunnel: w318 -> [w334 w335]
              tunnel: w315 -> [w332 _]
              tunnel: [w331 w335] -> w317
              tunnel: w313 -> [w327 _]
              tunnel: "The following .hawkeye files have been created:" ("string") -> [w324 _]
              frame False {
                w323 = "\n"  # Line Feed Constant
                w326 = "%s"  # format string
                # "Update the hawkeye created list"
                n130 = Array To Spreadsheet String(delimiter (Tab)=w323, array=w327, 3:w326) -> (spreadsheet string=w325:string)
                n131 = property class="Str"(reference=w332, error in=w334) -> (reference out=w329:refnum<vi>, error out=w333:errorcluster, "Value"=w330:string)
                n132 = Concatenate Strings(w330, w323, w324, w323, w323, w325, w323) -> (w328:string)
                n133 = property class="Str"(reference=w329, error in=w333, "Value"=w328) -> (error out=w331:errorcluster)  [unwired: 1 out]
              }
              frame True {
                # "No need to update any status"
              }
            }
          }
        }
      }
      frame "Generate HawkeyList" {
        # "Reset Generation/create Process"
        # "Regenerate Hawkeye List"
        n134 = Unbundle By Name(w344) -> ("Current Status Ref"=w338:refnum<vi>, "Generate HawkeyList?"=w341:bool, "Repository Path"=w337:path, "Status Indicator Ref"=w336:refnum<vi>)
        n135 = case "Generate Hawkey List?" shown="True" w341 {
          tunnel: [w345 w349] -> w343
          tunnel: w342 -> [w345 w348]
          tunnel: w338 -> [_ w350]
          tunnel: w337 -> [_ w347]
          tunnel: w336 -> [_ w346]
          frame False {
            # "Skipped Generate .Hawkey"
          }
          frame True {
            w352 = TRUE  # GUI Mode? {F)
            w351 = FALSE  # Check Changed Libraries Only?
            # "During Initial creation check all items in selected folder/path"
            # "Generate Hawkey List for selected LVLib / LVClass / Folder"
            n136 = call "UpdateActualDepsList.vi"("Overall Status Indicator Ref"=w346, "GUI Mode? {F)"=w352, "Current Status Indicator Ref"=w350, "error in (no error)"=w348, "UpdateForChangedLibrariesOnly"=w351, "Workspace Path"=w347) -> ("error out"=w349:errorcluster)  [unwired: 5 in]
          }
        }
        n137 = Bundle By Name(cluster=w344, "Generation Inprogress?"=FALSE) -> (w340:T1)
      }
      frame "Stop" {
        # "Performs actions when the VI is stopped."
        n138 = for {
          tunnel: string[] ["Exit"] -> [w359] mode=indexing
          shift-right: [w361] -> w356
          shift-left: w357 -> [w362]
          shift-right: [w358] -> _
          shift-left: w355 -> [w360]
          n139 = Enqueue Element(queue=w360, element=w359, error in (no error)=w362) -> (queue out=w358:refnum<queue>, error out=w361:errorcluster)  [unwired: 1 in, 1 out]
        }
      }
      frame "Exit" {
        w365 = TRUE  # Exit?
        # "Finish the execution"
        n140 = Release Queue(queue=w364, error in (no error)=w367) -> (error out=w363:errorcluster)  [unwired: 1 in, 2 out]
      }
      frame "Error" {
        # "Reset Process Status."
        # "In case of any Git API initialization errors, we need to disable the controls."
        # "Show the error dialog and clear out the operations. Update controls status."
        n141 = Current VI's Path() -> (path=w368:path)
        n142 = call "Error Logger.vi"("error in (no error)"=w370, "Current VI's Path"=w368) -> ("error out"=w369:errorcluster)  [unwired: 9 in]
        n143 = Flush Queue(queue=w377, error in (no error)=w369) -> (queue out=w374:refnum<queue>, error out=w375:errorcluster)  [unwired: 1 out]
        n144 = for {
          tunnel: string[] ["Enable Disable Controls"] -> [w380] mode=indexing
          shift-right: [w382] -> w373
          shift-left: w375 -> [w383]
          shift-right: [w379] -> _
          shift-left: w374 -> [w381]
          n145 = Enqueue Element(queue=w381, element=w380, error in (no error)=w383) -> (queue out=w379:refnum<queue>, error out=w382:errorcluster)  [unwired: 1 in, 1 out]
        }
        n146 = Bundle By Name(cluster=w378, "Generation Inprogress?"=FALSE) -> (w372:T1)
      }
    }
  }
  n147 = invoke class="VI" method="FP.Close"(error in=w3) -> (error out=w2:errorcluster)  [unwired: 2 in, 2 out]
  n148 = call <vilib>:"Clear Errors.vi"("error in (no error)"=w2) -> ()  [unwired: 5 in, 2 out]
